vi "Get Pane Details.vi"(8 "error in (no error)":errorcluster, 9 "Front Panel.ShowMenuBar":bool, 10 "Scale Factor":dbl, 11 "Panes[]":refnum<vi>[](array[refnum])) -> (0 "error out":errorcluster, 3 "Pane Details":T1[](array[typedef]))   [LabVIEW 2018]
uses:
  Typedefs/Pane Details--Cluster.ctl
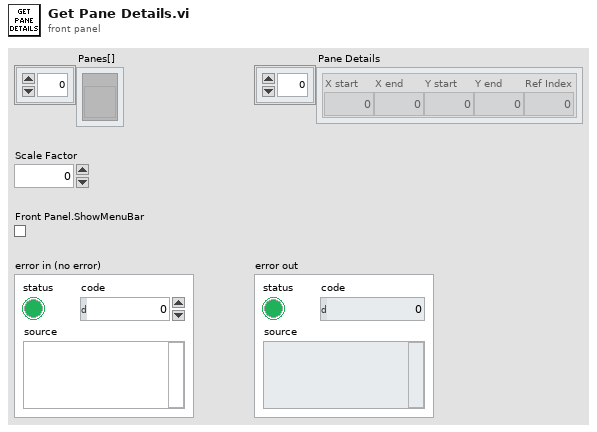
[diagram p1: front panel]
types:
  T1 = typedef "Pane Details--Cluster.ctl" = cluster{"X start":i32, "X end":i32, "Y start":i32, "Y end":i32, "Ref Index":i32}
  T2 = typedef "LVPointTypeDef.ctl" = cluster{"Horizontal":i16, "Vertical":i16}
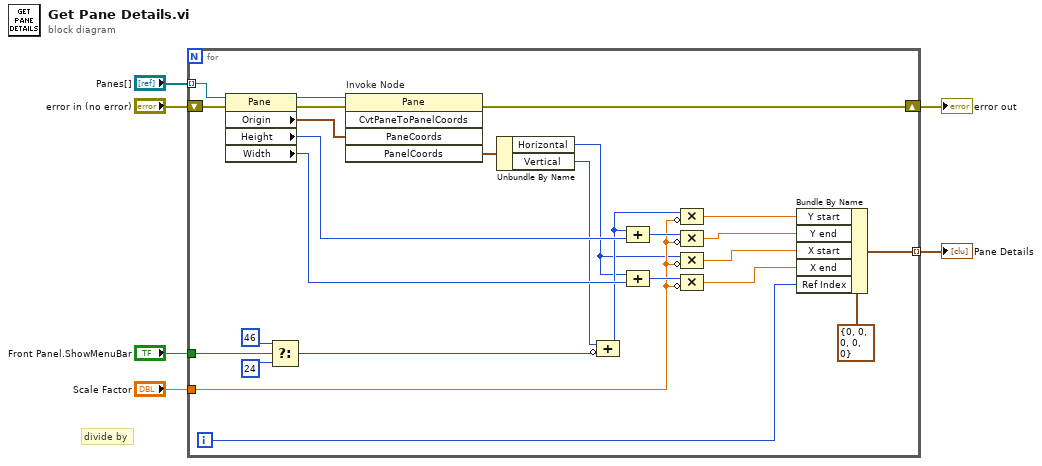
[diagram p0: block diagram]
diagram:
  # "divide by"
  n1 = for {
    tunnel: "Panes[]" -> [w32] mode=indexing
    tunnel: [w31] -> w4 mode=indexing
    tunnel: "Front Panel.ShowMenuBar" -> [w19]
    tunnel: "Scale Factor" -> [w24]
    shift-right: [w15] -> w1
    shift-left: "error in (no error)" -> [w30]
    i -> [w29]
    n2 = property class="Pane"(reference=w32, error in=w30) -> (reference out=w22:refnum<vi>, error out=w16:errorcluster, "Origin"=w14:T2, "Height"=w28:u32, "Width"=w27:u32)
    n3 = Select(t=46 ("value"), s=w19, f=24 ("value")) -> (s? t:f=w18:i32)
    n4 = invoke on="Invoke Node" class="Pane" method="CvtPaneToPanelCoords"(reference=w22, error in=w16, "PaneCoords"=w14) -> (error out=w15:errorcluster, "PanelCoords"=w11:T2)  [unwired: 2 in, 3 out]
    n5 = Unbundle By Name(w11) -> ("Horizontal"=w13:i16, "Vertical"=w12:i16)
    n6 = Compound Arithmetic op=unknown(w12, invert w18) -> (w17:i32)
    n7 = Compound Arithmetic op=ADD(w17, w28) -> (w26:u32)
    n8 = Compound Arithmetic op=ADD(w13, w27) -> (w25:u32)
    n9 = Compound Arithmetic op=MULTIPLY(w17, invert w24) -> (w9:dbl)
    n10 = Compound Arithmetic op=MULTIPLY(w26, invert w24) -> (w8:dbl)
    n11 = Compound Arithmetic op=MULTIPLY(w13, invert w24) -> (w7:dbl)
    n12 = Compound Arithmetic op=MULTIPLY(w25, invert w24) -> (w10:dbl)
    n13 = Bundle By Name(cluster=T1 {"X start"=0, "X end"=0, "Y start"=0, "Y end"=0, "Ref Index"=0}, "Y start"=w9, "Y end"=w8, "X start"=w7, "X end"=w10, "Ref Index"=w29) -> (w31:T1)
  }
  "Pane Details" <- w4
  "error out" <- w1
